vi "Index to Line Number.vi"(10 "Index":u32, 11 "Text":string) -> (2 "Line Count":u32, 3 "Line Number":u32)   [LabVIEW 2017]
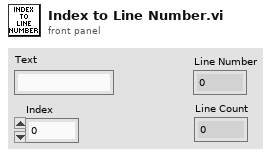
[diagram p1: front panel]
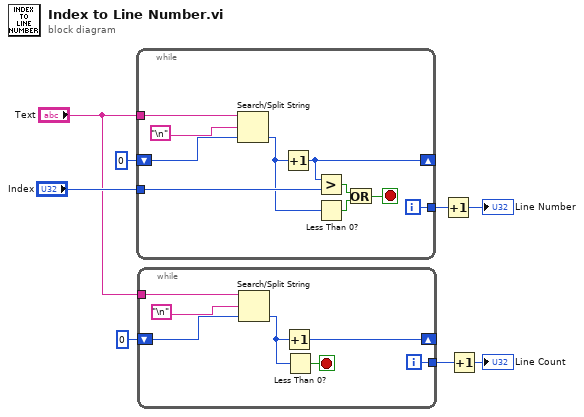
[diagram p0: block diagram]
diagram:
  n1 = while {
    tunnel: "Text" -> [w18]
    shift-right: [w13] -> _
    shift-left: 0 -> [w17]
    tunnel: [w16] -> w6
    tunnel: "Index" -> [w15]
    i -> [w16]
    stop <- w10 stop-if-true
    n2 = Search/Split String(string=w18, search string/char (-)="\n", offset (0)=w17) -> (offset of match=w9:i32)  [unwired: 2 out]
    n3 = Increment(x=w9) -> (x+1=w13:i32)
    n4 = Greater?(x=w13, y=w15) -> (0:w12:bool)
    n5 = Less Than 0?(x=w9) -> (x < 0?=w11:bool)
    n6 = Or(x=w12, y=w11) -> (x .or. y?=w10:bool)
  }
  n7 = while {
    tunnel: "Text" -> [w25]
    shift-right: [w21] -> _
    shift-left: 0 -> [w24]
    tunnel: [w23] -> w2
    i -> [w23]
    stop <- w19 stop-if-true
    n8 = Search/Split String(string=w25, search string/char (-)="\n", offset (0)=w24) -> (offset of match=w20:i32)  [unwired: 2 out]
    n9 = Increment(x=w20) -> (x+1=w21:i32)
    n10 = Less Than 0?(x=w20) -> (x < 0?=w19:bool)
  }
  n11 = Increment(x=w6) -> (x+1=→"Line Number":i32)
  n12 = Increment(x=w2) -> (x+1=→"Line Count":i32)
